vi "SW_Fire_TTL_at_start_stop.vi"(7 "TTL pulse length, ms":dbl=250.0 format="%#_13g", 8 "error in (no error)":errorcluster, 9 "Serial Port In":refnum<visa-resource-name>="COM3", 10 "Close VISA (T)":bool=TRUE, 11 "Start/stop signaling (F)":bool) -> (0 "error out":errorcluster, 1 "Serial Port Out":refnum<visa-resource-name>="COM3", 3 "Time spent to process command, ms":dbl=250.0)   [LabVIEW 2016]
doc: "Fires TTL High to the TTL2 output for ~250 ms (default)."
uses:
  <vilib>/Instr/_visa.llb/VISA Flush IO Buffer Mask.ctl
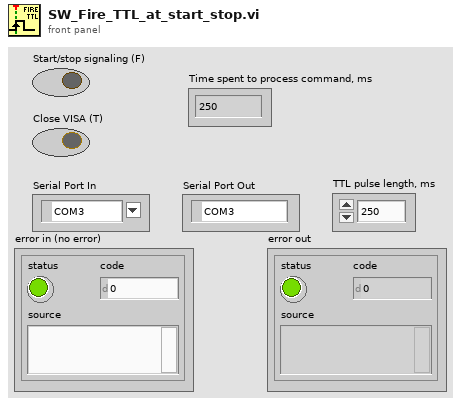
[diagram p1: front panel]
types:
  T1 = typedef "VISA Flush IO Buffer Mask.ctl" = u16
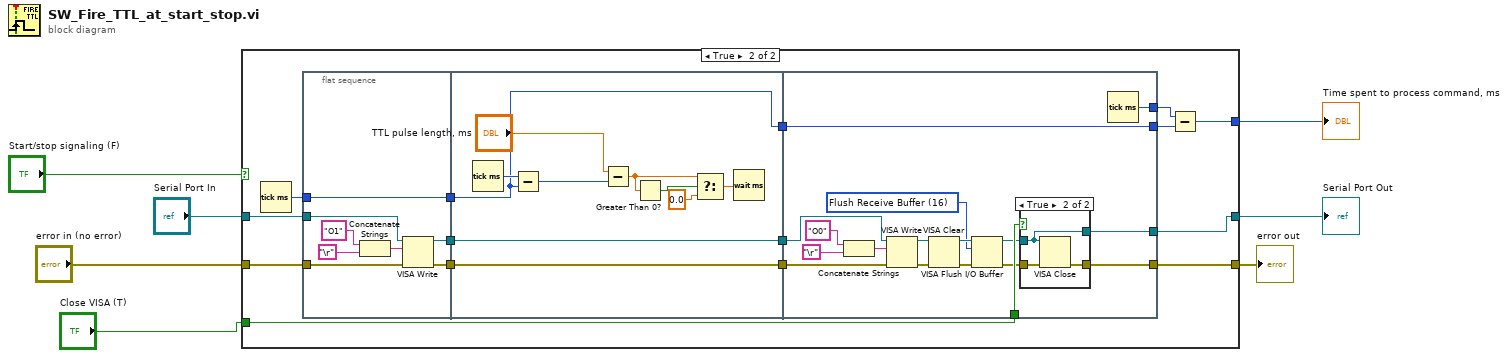
[diagram p0: block diagram]
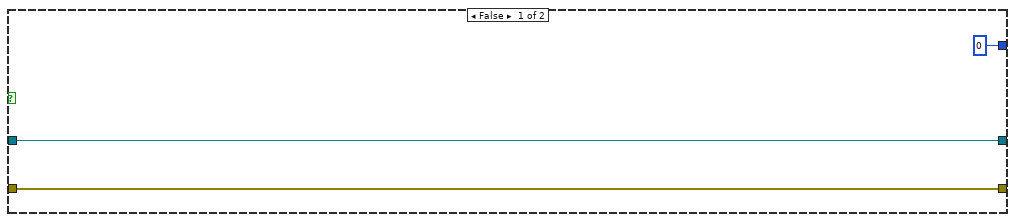
[diagram p2: hidden frame]
diagram:
  n1 = case shown="True" "Start/stop signaling (F)" {
    tunnel: [u32 0 w16] -> w7
    tunnel: [w9 w15] -> w6
    tunnel: "Serial Port In" -> [w9 w14]
    tunnel: "Close VISA (T)" -> [_ w13]
    tunnel: [w8 w12] -> w2
    tunnel: "error in (no error)" -> [w8 w11]
    frame False {
    }
    frame True {
      n2 = Tick Count (ms)() -> (millisecond timer value=w20:u32)
      n3 = flat-sequence {
        tunnel: w14 -> [w28]
        tunnel: [w30] -> w25
        tunnel: [w29] -> w24
        tunnel: [w27] -> w21
        tunnel: w20 -> [w27]
        tunnel: w11 -> [w26]
        tunnel: [w43] -> w23
        tunnel: w25 -> [w43]
        tunnel: [w42] -> w22
        tunnel: w24 -> [w42]
        tunnel: w21 -> [w34]
        tunnel: [w34] -> w17
        tunnel: [w57] -> w12
        tunnel: [w58] -> w15
        tunnel: [w59] -> w18
        tunnel: [w60] -> w19
        tunnel: w13 -> [w54]
        tunnel: w17 -> [w59]
        tunnel: w22 -> [w48]
        tunnel: w23 -> [w47]
        frame #0 {
          n4 = Concatenate Strings("O1" ("string"), "\r") -> (w33:string)
          n5 = VISA Write(VISA resource name=w28, write buffer=w33, error in (no error)=w26) -> (VISA resource name out=w30:refnum<visa-resource-name>, error out=w29:errorcluster)  [unwired: 1 out]
        }
        frame #1 {
          n6 = Tick Count (ms)() -> (millisecond timer value=w41:u32)
          n7 = Subtract(x=w41, y=w34) -> (x-y=w39:u32)
          n8 = Subtract(x="TTL pulse length, ms", y=w39) -> (x-y=w36:dbl)
          n9 = Greater Than 0?(x=w36) -> (x > 0?=w38:bool)
          n10 = Select(t=w36, s=w38, f=0.0) -> (s? t:f=w37:dbl)
          n11 = Wait (ms)(milliseconds to wait=w37) -> ()  [unwired: 1 out]
        }
        frame #2 {
          w49 = T1 16 items=["Flush Receive Buffer"=16, "Write Transmit Buffer to Device"=32, "Flush Receive Buffer (No I/O)"=64, "Flush Transmit Buffer"=128] ("Mask")
          n12 = Concatenate Strings("O0" ("string"), "\r") -> (w46:string)
          n13 = VISA Write(VISA resource name=w47, write buffer=w46, error in (no error)=w48) -> (VISA resource name out=w45:refnum<visa-resource-name>, error out=w44:errorcluster)  [unwired: 1 out]
          n14 = VISA Clear(VISA resource name=w45, error in (no error)=w44) -> (VISA resource name out=w51:refnum<visa-resource-name>, error out=w53:errorcluster)
          n15 = VISA Flush I/O Buffer(VISA resource name=w51, mask (16)=w49, error in (no error)=w53) -> (VISA resource name out=w50:refnum<visa-resource-name>, error out=w52:errorcluster)
          n16 = case shown="True" w54 {
            tunnel: w50 -> [w62 w64]
            tunnel: w52 -> [w61 w63]
            tunnel: [w62 w64] -> w58
            tunnel: [w61 w65] -> w57
            frame False {
            }
            frame True {
              n17 = VISA Close(VISA resource name=w64, error in (no error)=w63) -> (error out=w65:errorcluster)
            }
          }
          n18 = Tick Count (ms)() -> (millisecond timer value=w60:u32)
        }
      }
      n19 = Subtract(x=w19, y=w18) -> (x-y=w16:u32)
    }
  }
  "Time spent to process command, ms" <- w7
  "Serial Port Out" <- w6
  "error out" <- w2
